vi "load_hardware_ini.vi"(9 "name or relative path":string, 10 "Application Directory":path) -> (2 "Available stages":string[](array[string]), 3 "Available cameras":string[](array[string]))   [LabVIEW 2018]
uses:
  <vilib>/Utility/config.llb/Read Key (String).vi
  <vilib>/Utility/config.llb/NI_LVConfig.lvlib
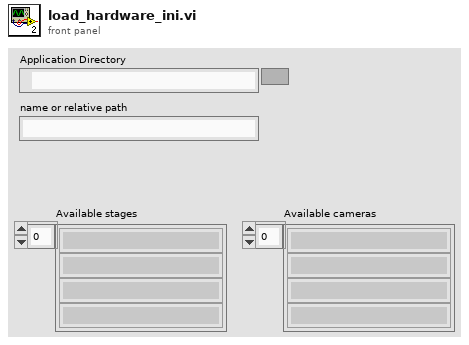
[diagram p1: front panel]
types:
  T1 = typedef "NI_LVConfig.lvlib/Config Data RefNum.ctl" = refnum<k1>
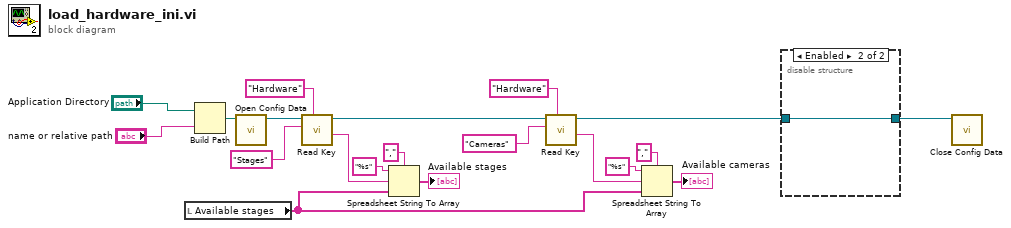
[diagram p0: block diagram]
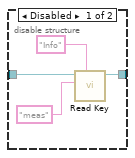
[diagram p2: hidden frame]
diagram:
  n1 = local read "Available stages"() -> (w1:string[])
  n2 = Build Path(base path="Application Directory", name or relative path="name or relative path") -> (appended path=w5:path)
  n3 = call <vilib>:"Open Config Data.vi"("configuration file path"=w5) -> ("refnum"=w6:T1)  [unwired: 8 in, 2 out]
  n4 = call-poly <vilib>:"Read Key.vi"("section"="Hardware", "key"="Stages", "refnum"=w6) -> ("value"=w11:string, "refnum out"=w19:T1)  [unwired: 5 in, 2 out]
  n5 = Spreadsheet String To Array(delimiter (Tab)=",", format string="%s", spreadsheet string=w11, array type (2D Dbl)=w1) -> (array=→"Available stages":string[])
  n6 = call-poly <vilib>:"Read Key.vi"("section"="Hardware", "key"="Cameras", "refnum"=w19) -> ("value"=w17:string, "refnum out"=w20:T1)  [unwired: 5 in, 2 out]
  n7 = Spreadsheet String To Array(delimiter (Tab)=",", format string="%s", spreadsheet string=w17, array type (2D Dbl)=w1) -> (array=→"Available cameras":string[])
  n8 = disable-structure shown="Enabled" {
    disable-tunnel: w20 -> [w24 w25]
    disable-tunnel: [w23 w25] -> w2
    frame Disabled {
      n9 = call-poly <vilib>:"Read Key.vi"("section"="Info", "key"="meas", "refnum"=w24) -> ("refnum out"=w23:T1)  [unwired: 5 in, 3 out]
    }
    frame Enabled {
    }
  }
  n10 = call <vilib>:"Close Config Data.vi"("refnum"=w2) -> ()  [unwired: 9 in, 2 out]
